vi "Form Error Message.vi"(0 "Error Message":string[](array[string]), 1 "error code (0)":i32, 2 "Error?":bool, 11 "error in (no error)":errorcluster) -> (15 "error out":errorcluster)   [LabVIEW 2024]
uses:
  4da3fa3f-d6a2-4c6b-9c9c-fc44bca91f7b.vi
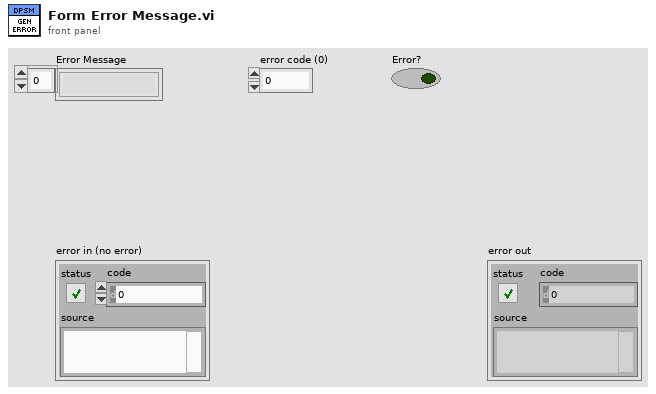
[diagram p1: front panel]
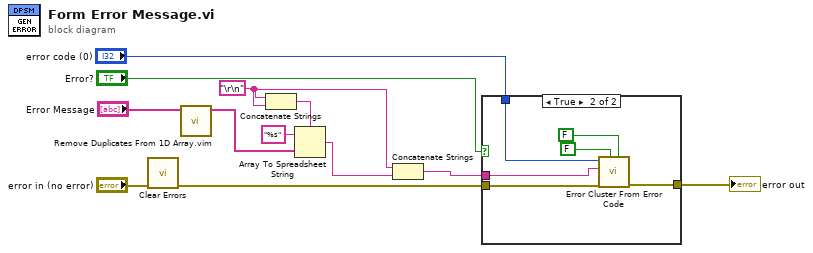
[diagram p0: block diagram]
diagram:
  w2 = "\r\n"
  n1 = call <vilib>:"Clear Errors.vi"("error in (no error)"="error in (no error)") -> ("error out"=w4:errorcluster)  [unwired: 5 in, 1 out]
  n2 = call "Remove Duplicates From 1D Array.vim"("array"="Error Message") -> ("array with duplicates removed"=w7:string[])  [unwired: 10 in]
  n3 = Concatenate Strings(w2, w2) -> (w1:string)
  n4 = Array To Spreadsheet String(delimiter (Tab)=w1, array=w7, 3:"%s" ("format string")) -> (spreadsheet string=w5:string)
  n5 = Concatenate Strings(w2, w5) -> (w3:string)
  n6 = case shown="True" "Error?" {
    tunnel: w4 -> [w13 w19]
    tunnel: [w13 w18] -> w11
    tunnel: w3 -> [_ w17]
    tunnel: "error code (0)" -> [_ w15]
    frame False {
    }
    frame True {
      n7 = call <vilib>:"Error Cluster From Error Code.vi"("is warning? (False)"=FALSE, "show call chain? (False)"=FALSE, "error in (no error)"=w19, "error message (\"\")"=w17, "error code (0)"=w15) -> ("error out"=w18:errorcluster)  [unwired: 4 in]
    }
  }
  "error out" <- w11
